vi "Mask Write Holding Register.vi"(4 "OR mask":u16, 6 "AND mask":u16, 8 "error in (no error)":errorcluster, 10 "address":u16, 11 "Modbus master in":refnum<class "Network Master.lvclass">) -> (0 "error out":errorcluster, 3 "Modbus master out":refnum<class "Network Master.lvclass">)   [LabVIEW 2021, in "Network Master.lvclass"]
doc: "Writes values to one or more bits of a holding register."
uses:
  Network Master.lvclass
  D:/my_projects/projects/Algorithms/Labview/21/Modbus_v121c/Network Protocol/Network Protocol.lvclass
  Modbus Data Unit/Modbus Data Unit.lvclass/Modbus Data Unit.ctl
  Network Protocol.lvclass/Network Protocol.ctl
  Network Master.lvclass/Network Master.ctl
  Read Transmission Data Unit.vi
  Modbus Data Unit/Construct PDU.vi
  Master Function Definition/Function code mismatch error.vi
  Data Model/Error Generator.vi
  Modbus Data Unit/Deconstruct PDU.vi
  Modbus Data Unit/Modbus Data Unit.lvclass
  Transmission Data Unit/Transmission Data Unit.lvclass
  Master Function Definition/Master Function Definition.lvclass
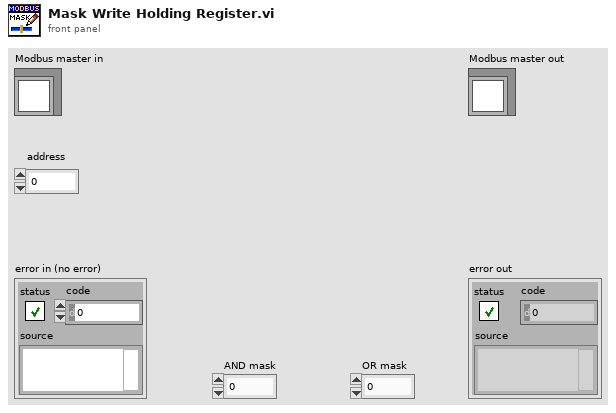
[diagram p1: front panel]
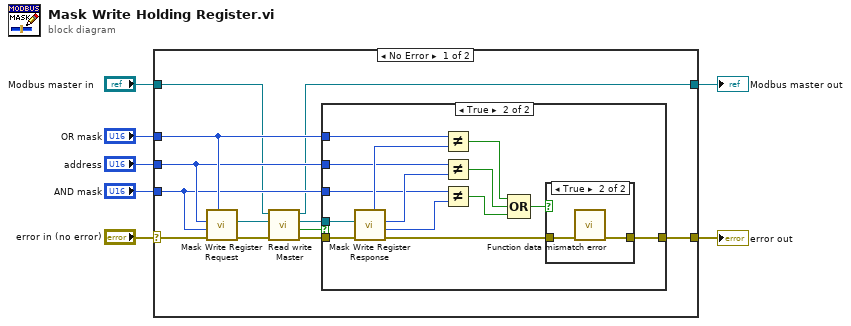
[diagram p0: block diagram]
diagram:
  n1 = case shown="No Error" "error in (no error)" {
    selector: "error in (no error)" -> [w8 w38]
    tunnel: "Modbus master in" -> [w9 w39]
    tunnel: [w10 w39] -> w6
    tunnel: [w18 w38] -> w5
    tunnel: "OR mask" -> [w16 _]
    tunnel: "address" -> [w15 _]
    tunnel: "AND mask" -> [w14 _]
    frame No Error {
      n2 = call "Mask Write Register Request.vi"("OR mask"=w16, "error in"=w8, "AND mask"=w14, "Starting Address"=w15) -> ("error out"=w19:errorcluster, "modbus data unit out"=w13:refnum<class "Modbus Data Unit.lvclass">)  [unwired: 6 in]
      n3 = call "Read write Master.vi"("error in (no error)"=w19, "Modbus data unit in"=w13, "Modbus master in"=w9) -> ("error out"=w17:errorcluster, "PDU valid?"=w12:bool, "Modbus data unit out"=w11:refnum<class "Modbus Data Unit.lvclass">, "Modbus master out"=w10:refnum<class "Network Master.lvclass">)  [unwired: 5 in]
      n4 = case shown="True" w12 {
        tunnel: [w20 w32] -> w18
        tunnel: w17 -> [w20 w29]
        tunnel: w11 -> [_ w28]
        tunnel: w16 -> [_ w23]
        tunnel: w14 -> [_ w22]
        tunnel: w15 -> [_ w21]
        frame False {
        }
        frame True {
          n5 = call "Mask Write Register Response.vi"("error in"=w29, "modbus data unit in"=w28) -> ("error out"=w27:errorcluster, "AND mask"=w30:u16, "Address"=w31:u16, "OR mask"=w24:u16)  [unwired: 6 in]
          n6 = Not Equal?(x=w23, y=w24) -> (x != y?=w25:bool)
          n7 = Not Equal?(x=w21, y=w31) -> (x != y?=w26:bool)
          n8 = Not Equal?(x=w22, y=w30) -> (x != y?=w34:bool)
          n9 = Compound Arithmetic op=OR(w25, w26, w34) -> (w33:bool)
          n10 = case shown="True" w33 {
            tunnel: [w35 w37] -> w32
            tunnel: w27 -> [w35 w36]
            frame False {
            }
            frame True {
              n11 = call "Function data mismatch error.vi"("error in (no error)"=w36) -> ("error out"=w37:errorcluster)  [unwired: 10 in]
            }
          }
        }
      }
    }
    frame Error {
    }
  }
  "error out" <- w5
  "Modbus master out" <- w6
